vi "Normalise holo.vi"(1 "holo _comb in":dbl[](array[numeric])) -> (0 "holo_comb out":u8[](array[numeric]))   [LabVIEW 2020]
uses:
  _globals/OpticalPrime Controls.vi
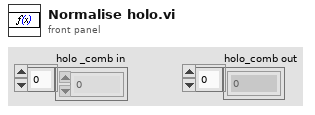
[diagram p1: front panel]
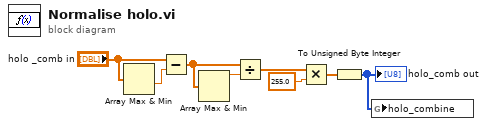
[diagram p0: block diagram]
diagram:
  n1 = Array Max & Min(array="holo _comb in") -> (min value=w4:dbl)  [unwired: 3 out]
  n2 = Subtract(x="holo _comb in", y=w4) -> (x-y=w5:dbl[])
  n3 = Array Max & Min(array=w5) -> (max value=w6:dbl)  [unwired: 3 out]
  n4 = Divide(x=w5, y=w6) -> (x/y=w7:dbl[])
  n5 = Multiply(x=w7, y=255.0) -> (x*y=w3:dbl[])
  n6 = To Unsigned Byte Integer(number=w3) -> (unsigned 8bit integer=w1:u8[])
  "holo_comb out" <- w1
  n7 = global write "OpticalPrime Controls.vi" "holo_combine"(w1) -> ()
